vi "Close.vi"(8 "error in (no error)":errorcluster, 11 "RTL-SDR in":refnum<class "RTL-SDR.lvclass">) -> (0 "error out":errorcluster, 1 "function return":i32, 3 "RTL-SDR out":refnum<class "RTL-SDR.lvclass">)   [LabVIEW 2015, in "RTL-SDR.lvclass"]
doc: "Created IvanLis by LabVIEW Portal\nProfile: http://labviewportal.org/memberlist.php?mode=viewprofile&u=987\neMail: IvanLisanov@gMail.com\nTelegram: https://t.me/IvanLis"
uses:
  RTL-SDR.lvclass
  RTL-SDR.lvclass/RTL-SDR.ctl
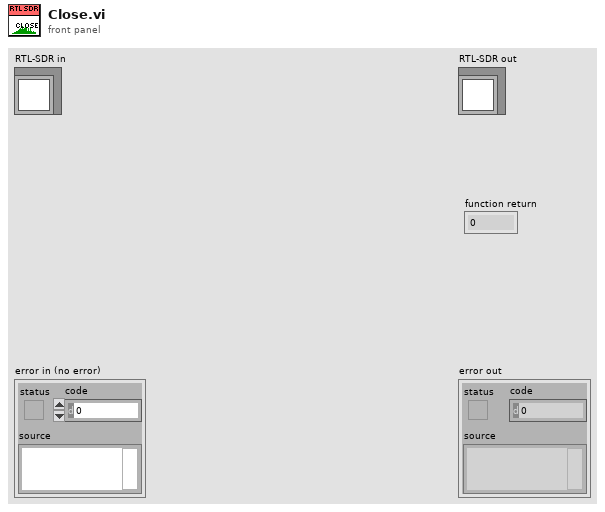
[diagram p1: front panel]
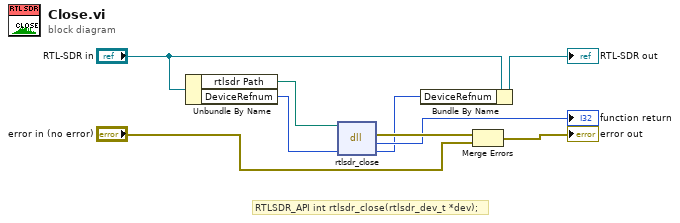
[diagram p0: block diagram]
diagram:
  # "RTLSDR_API int rtlsdr_close(rtlsdr_dev_t *dev);"
  n1 = Unbundle By Name("RTL-SDR in") -> ("rtlsdr Path"=w5:path, "DeviceRefnum"=w4:u64)
  n2 = dll-call lib="C:/Users/Ivan/Desktop/D-23-09-24 (RTL-SDR)/Project (Pelleng-SDR)/rtlsdr/dll/rtlsdr.dll" fn="rtlsdr_close"(path in=w5, "DeviceRefnum"=w4) -> (error out=w9:errorcluster, "return type"=→"function return":i32, "DeviceRefnum"=w3:u64)  [unwired: 2 in, 1 out]
  n3 = Bundle By Name(cluster="RTL-SDR in", "DeviceRefnum"=w3) -> (→"RTL-SDR out":refnum<class "RTL-SDR.lvclass">)
  n4 = Merge Errors(w9, "error in (no error)") -> (→"error out":errorcluster)
